vi "orderDefRobots.vi"(8 "error in (no error)":errorcluster, 9 "Array of Robots":refnum<class "Robot.lvclass">[](array[class]), 10 "Game":refnum<class "Game.lvclass">, 11 "Utilities in":refnum<class "Utilities.lvclass">) -> (0 "error out":errorcluster, 2 "Odered array of robots":dbl[][](array[numeric]), 3 "Utilities out":refnum<class "Utilities.lvclass">)   [LabVIEW 2023, in "Utilities.lvclass"]
uses:
  Utilities.lvclass
  Game_class/Game.lvclass
  Robot_class/Robot.lvclass
  Game_class/Game.lvclass/Game.ctl
  Object_class/Object.lvclass/Object.ctl
  Robot_class/Robot.lvclass/Robot.ctl
  Object_class/Read x.vi
  Object_class/Read y.vi
  Robot_class/Read id.vi
  cbccac48-48e3-4c62-8aed-d79219be0951.vi
  Game_class/Read FieldRef.vi
  <vilib>/Array/Sort 2D Array - Pop Stack.vi
  <vilib>/Array/Sort 2D Array - Push Stack.vi
  cbccac48-48e3-4c62-8aed-d79219be0951.vi/269d4b3b-47f5-49e3-8884-44851e4dd9d5.vi
  cbccac48-48e3-4c62-8aed-d79219be0951.vi/6d99389c-673d-4efb-bf33-19b32bcf4cf8.vi
  Field_class/Field.lvclass
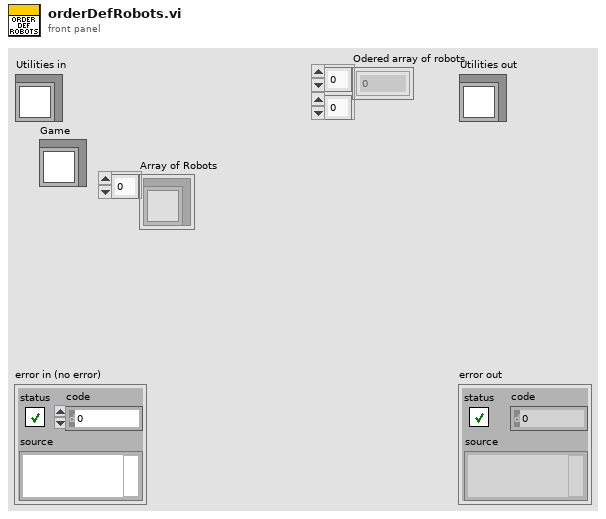
[diagram p1: front panel]
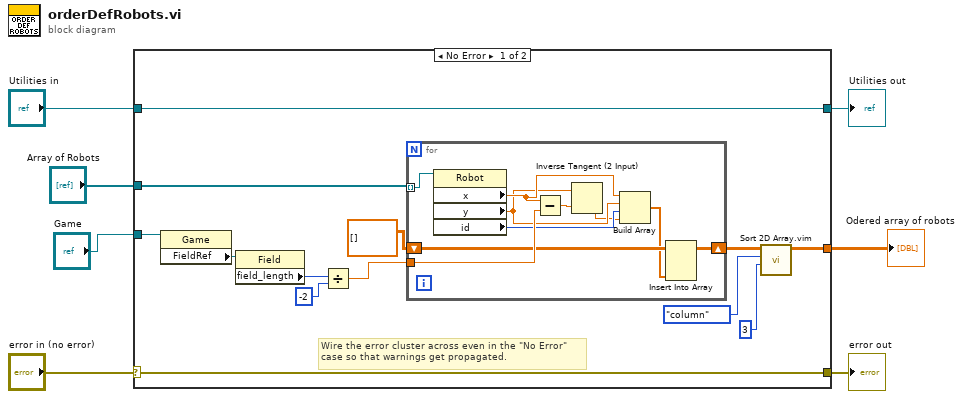
[diagram p0: block diagram]
diagram:
  n1 = case shown="No Error" "error in (no error)" {
    selector: "error in (no error)" -> [w19 w32]
    tunnel: [w19 w32] -> w6
    tunnel: [w20 w31] -> w4
    tunnel: "Utilities in" -> [w20 w31]
    tunnel: "Array of Robots" -> [w18 _]
    tunnel: "Game" -> [w17 _]
    tunnel: [w8 _] -> w1
    frame No Error {
      # "Wire the error cluster across even in the \"No Error\"\ncase so that warnings get propagated."
      n2 = property class="Game"(reference=w17) -> ("FieldRef"=w16:refnum<class "Field.lvclass">)  [unwired: 1 in, 2 out]
      n3 = property class="Field"(reference=w16) -> ("field_length"=w15:i32)  [unwired: 1 in, 2 out]
      n4 = Divide(x=w15, y=-2) -> (x/y=w13:dbl)
      n5 = for {
        tunnel: w18 -> [w30] mode=indexing
        tunnel: w13 -> [w29]
        shift-right: [w27] -> w11
        shift-left: dbl[][] [] -> [w28]
        n6 = property class="Robot"(reference=w30) -> ("x"=w25:dbl, "y"=w24:dbl, "id"=w23:i32)  [unwired: 1 in, 2 out]
        n7 = Subtract(x=w25, y=w29) -> (x-y=w26:dbl)
        n8 = Inverse Tangent (2 Input)(1:w26, 2:w24) -> (0:w22:dbl)
        n9 = Build Array(w25, w24, w23, w22) -> (w21:dbl[])
        n10 = Insert Into Array(array=w28, new element=w21) -> (w27:dbl[][])  [unwired: 2 in]
      }
      n11 = call "Sort 2D Array.vim"("index"=3, "dimension to index (column)"=enum16{"column", "row"}."column", "2D array"=w11) -> ("sorted 2D array"=w8:dbl[][])  [unwired: 7 in, 1 out]
    }
    frame Error {
    }
  }
  "error out" <- w6
  "Utilities out" <- w4
  "Odered array of robots" <- w1
